vi "Read_Txt_File.vi"(3 "error in (no error)":errorcluster, 5 "Path":path) -> (0 "error out":errorcluster, 2 "Text":string)   [LabVIEW 2023]
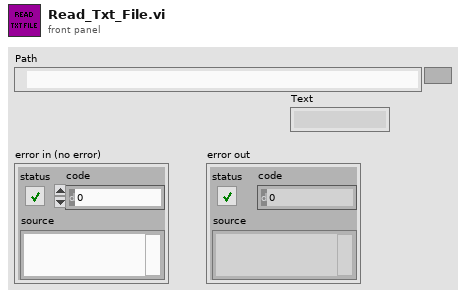
[diagram p1: front panel]
types:
  T1 = enum16{"open", "replace", "create", "open or create", "replace or create", "replace or create with confirmation"}
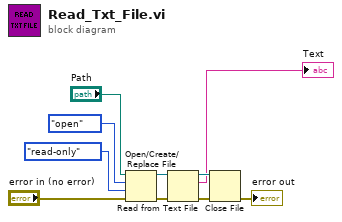
[diagram p0: block diagram]
diagram:
  n1 = Open/Create/Replace File(file path (use dialog)="Path", error in="error in (no error)", operation (0:open)=T1."open", access (0:read/write)=enum16{"read/write", "read-only", "write-only"}."read-only") -> (refnum out=w8:refnum<file>, error out=w3:errorcluster)  [unwired: 2 in, 1 out]
  n2 = Read from Text File(file (use dialog)=w8, error in=w3) -> (refnum out=w10:refnum<file>, text=→"Text":string, error out=w7:errorcluster)  [unwired: 2 in, 1 out]
  n3 = Close File(refnum=w10, error in=w7) -> (error out=→"error out":errorcluster)  [unwired: 1 out]
